vi "DAQ@ChannelName__Parameter.vi"(1 "ParamterIn":string) -> (0 "ParamterOut":string)   [LabVIEW 2019]
panel:
  in  "ChannelName":string(combo)
  in  "DAQName":string(combo)
  in  "Confirm":bool
  # "DAQ@ChannelName $DAQ,$ChannelName1,$ChannelName2....."
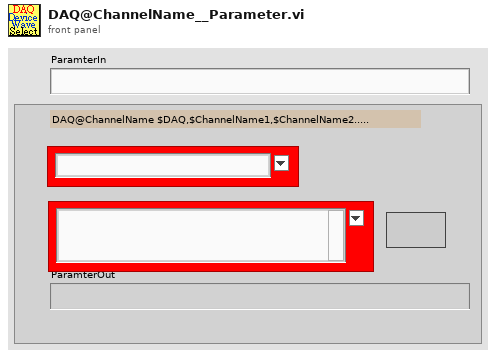
[diagram p1: front panel]
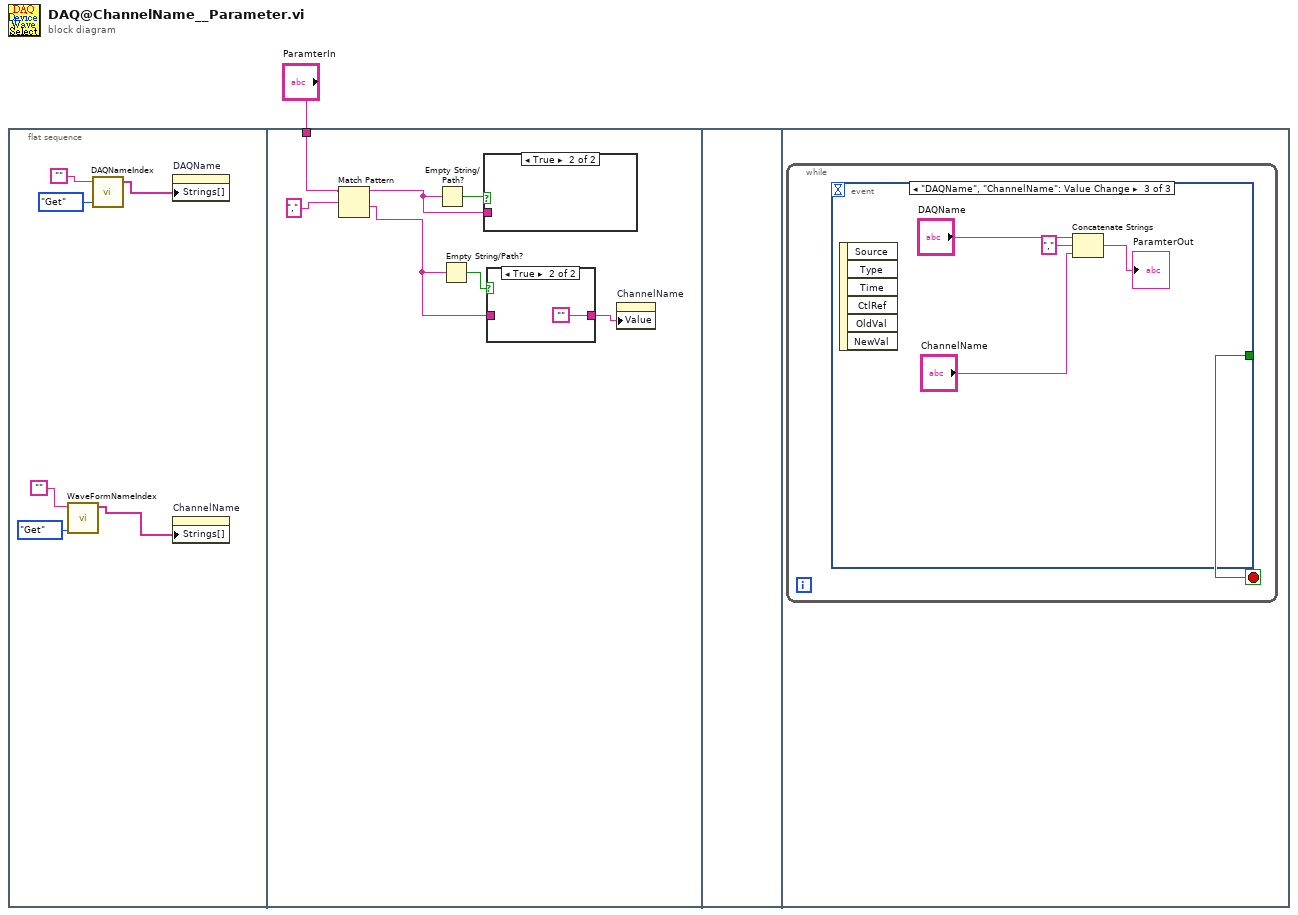
[diagram p0: block diagram]
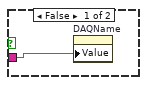
[diagram p3: hidden frame]
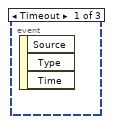
[diagram p4: hidden frame]
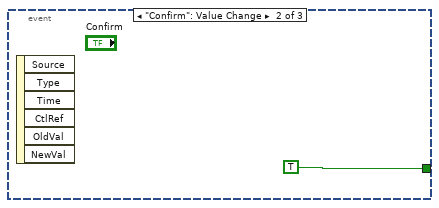
[diagram p5: hidden frame]
diagram:
  n1 = flat-sequence {
    tunnel: "ParamterIn" -> [w11]
    frame #0 {
      n2 = call "WaveFormNameIndex.vi"("OP"=enum16{"Get", "Update", "Init", "GetSPS"}."Get", "WaveFormName"="") -> ("WaveFormNameList"=w2:string[])  [unwired: 6 in, 3 out]
      n3 = call "DAQNameIndex.vi"("OP"=enum16{"Get", "Update", "Init"}."Get", "DAQName"="") -> ("DAQList"=w5:string[])  [unwired: 1 in, 2 out]
      n4 = property on="DAQName" class="CmbBox"("Strings[]"=w5) -> ()  [unwired: 2 in, 2 out]
      n5 = property on="ChannelName" class="CmbBox"("Strings[]"=w2) -> ()  [unwired: 2 in, 2 out]
    }
    frame #1 {
      n6 = Match Pattern(string=w11, regular expression="," ("search string/char (-)")) -> (before substring=w9:string, after substring=w8:string)  [unwired: 1 in, 2 out]
      n7 = Empty String/Path?(string/path=w9) -> (empty?=w14:bool)
      n8 = Empty String/Path?(string/path=w8) -> (empty?=w13:bool)
      n9 = case shown="True" w14 {
        tunnel: w9 -> [w17 _]
        frame False {
          n10 = property on="DAQName" class="CmbBox"("Value"=w17) -> ()  [unwired: 2 in, 2 out]
        }
        frame True {
        }
      }
      n11 = case shown="True" w13 {
        tunnel: [w15 ""] -> w12
        tunnel: w8 -> [w15 _]
        frame False {
        }
        frame True {
        }
      }
      n12 = property on="ChannelName" class="CmbBox"("Value"=w12) -> ()  [unwired: 2 in, 2 out]
    }
    frame #2 {
    }
    frame #3 {
      n13 = while {
        stop <- w18 stop-if-true
        n14 = event shown="[2] \"DAQName\", \"ChannelName\": Value Change" {
          selector: _ -> [_ _ _]
          dyn-events: _ -> [_ _ _]
          timeout: _ -> [_ _ _]
          tunnel: [_ TRUE _] -> w18
          event Timeout {
            n15 = event-data() -> ()  [unwired: 1 in, 3 out]
          }
          event "Confirm": Value Change {
            n16 = event-data() -> ()  [unwired: 1 in, 6 out]
          }
          event "DAQName", "ChannelName": Value Change {
            n17 = event-data() -> ()  [unwired: 1 in, 6 out]
            n18 = Concatenate Strings("DAQName", "," ("string"), "ChannelName") -> (→"ParamterOut":string)
          }
        }
      }
    }
  }
